vi "average Y.vi"() -> ()   [LabVIEW 2011]
panel:
  in  "click":bool
  in  "average Z":dbl
  in  "average X":dbl
  in  "average Y":dbl
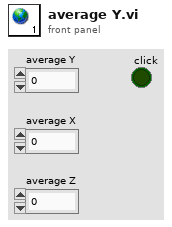
[diagram p1: front panel]
diagram:
